vi "Create Color Object.vi"(8 "Error In":errorcluster, 11 "Color (black)":u32(colorbox)) -> (0 "Error Out":errorcluster, 3 "Color Object":refnum<k24>)   [LabVIEW 2020, in "Dot Net UI Controls.lvlib"]
uses:
  Dot Net UI Controls.lvlib
  System.Drawing
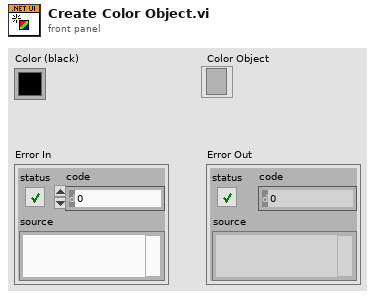
[diagram p1: front panel]
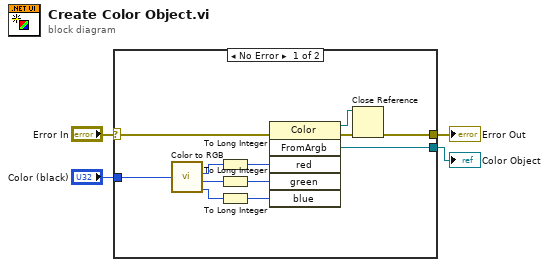
[diagram p0: block diagram]
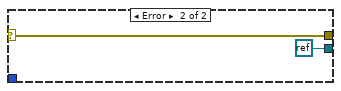
[diagram p2: hidden frame]
diagram:
  n1 = case shown="No Error" "Error In" {
    selector: "Error In" -> [w5 w18]
    tunnel: [w16 w18] -> w2
    tunnel: "Color (black)" -> [w13 _]
    tunnel: [w12 refnum<k0> refnum] -> w3
    frame No Error {
      n2 = call <vilib>:"Color to RGB.vi"("Color"=w13) -> ("R"=w7:u8, "G"=w6:u8, "B"=w10:u8)  [unwired: 1 out]
      n3 = To Long Integer(number=w7) -> (32bit integer=w8:i32)
      n4 = To Long Integer(number=w6) -> (32bit integer=w9:i32)
      n5 = To Long Integer(number=w10) -> (32bit integer=w11:i32)
      n6 = invoke class="Color" method="FromArgb"(error in=w5, "red"=w8, "green"=w9, "blue"=w11) -> (reference out=w15:refnum<k24>, error out=w14:errorcluster, "FromArgb"=w12:refnum<k24>)  [unwired: 2 in, 3 out]
      n7 = Close Reference(reference=w15, error in (no error)=w14) -> (error out=w16:errorcluster)
    }
    frame Error {
    }
  }
  "Color Object" <- w3
  "Error Out" <- w2
